vi "Read.vi"(11 "HighLimit Condition Config in":refnum<class "HighLimit Condition Config.lvclass">) -> (2 "Limit":dbl, 3 "Source":string)   [LabVIEW 2020, in "VolatusSeqConfig.lvlib" / "HighLimit Condition Config.lvclass"]
uses:
  HighLimit Condition Config.lvclass
  HighLimit Condition Config.lvclass/HighLimit Condition Config.ctl
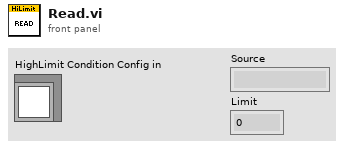
[diagram p1: front panel]
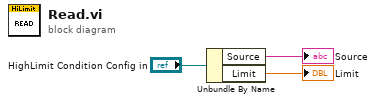
[diagram p0: block diagram]
diagram:
  n1 = Unbundle By Name("HighLimit Condition Config in") -> ("Source"=→"Source":string, "Limit"=→"Limit":dbl)
